vi "Get_Maximal_Length_of_Subtracks-1.vi"(1 "[IN] Subtracks":T1(array[cluster])) -> (0 "[OUT] Maximal Length":i32)   [LabVIEW 2013]
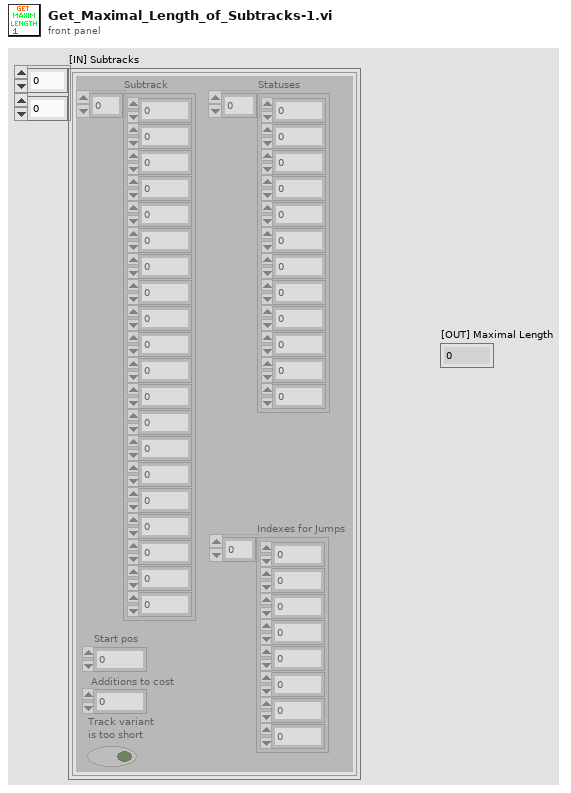
[diagram p1: front panel]
types:
  T1 = cluster{"Subtrack":dbl[], "Statuses":i16[], "Start pos":i32, "Additions to cost":i32, "Track variant \nis too short":bool, "Indexes for Jumps":i32[]}[][]
  T2 = cluster{"Subtrack":dbl[], "Statuses":i16[], "Start pos":i32, "Additions to cost":i32, "Track variant \nis too short":bool, "Indexes for Jumps":i32[]}[]
  T3 = cluster{"Subtrack":dbl[], "Statuses":i16[], "Start pos":i32, "Additions to cost":i32, "Track variant \nis too short":bool, "Indexes for Jumps":i32[]}
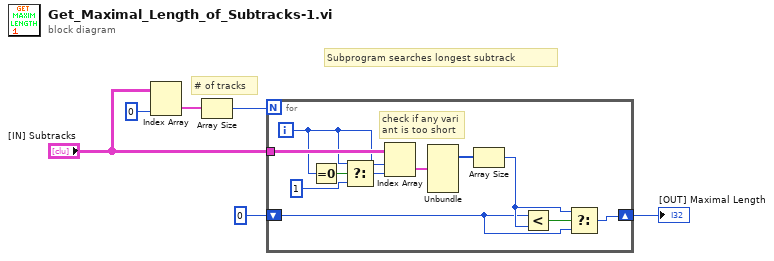
[diagram p0: block diagram]
diagram:
  # "Subprogram searches longest subtrack"
  # "# of tracks"
  n1 = Index Array(array="[IN] Subtracks", index (col)=0 ("disabled index (col)")) -> (element=w6:T2)  [unwired: 1 in]
  n2 = Array Size(array=w6) -> (size(s)=w4:i32)
  n3 = for {
    N: w4 -> [_]
    tunnel: "[IN] Subtracks" -> [w17]
    shift-right: [w8] -> w1
    shift-left: 0 -> [w9]
    i -> [w12]
    # "check if any vari\nant is too short"
    n4 = Equal To 0?(x=w12) -> (x = 0?=w15:bool)
    n5 = Select(t=w12, s=w15, f=1) -> (s? t:f=w13:i32)
    n6 = Index Array(array=w17, index (row)=w12, index (col)=w13) -> (element=w16:T3)
    n7 = Unbundle(w16) -> ("Statuses"=w7:i16[])  [unwired: 5 out]
    n8 = Array Size(array=w7) -> (size(s)=w10:i32)
    n9 = Less?(x=w9, y=w10) -> (x < y?=w11:bool)
    n10 = Select(t=w10, s=w11, f=w9) -> (s? t:f=w8:i32)
  }
  "[OUT] Maximal Length" <- w1
